vi "EJ 3.3.vi"() -> ()   [LabVIEW 2013]
uses:
  <vilib>/sound2/lvsound2.llb/Sound Input Read (DBL).vi
panel:
  in  "stop":bool
  in  "Cluster":T1
  out "Waveform Graph":dbl[](graph)
  in  "Buffer de lectura":dbl=11025.0
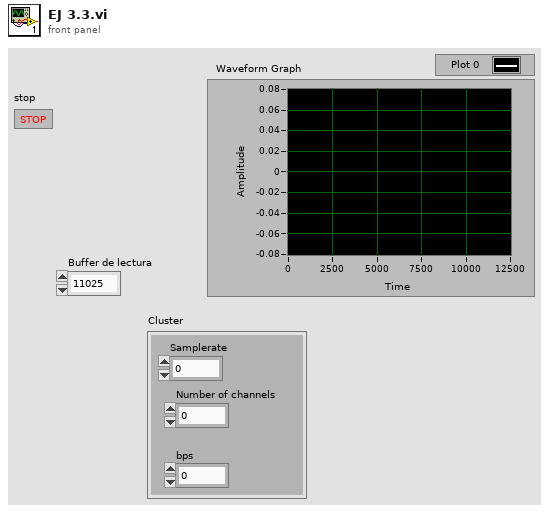
[diagram p1: front panel]
types:
  T1 = cluster{"Samplerate":dbl, "Number of channels":dbl, "bps":dbl}
  T2 = typedef "Sound Input Task ID.ctl" = u32
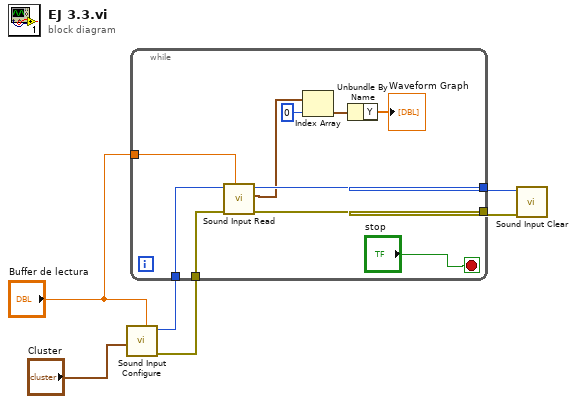
[diagram p0: block diagram]
diagram:
  n1 = call <vilib>:"Sound Input Configure.vi"("number of samples/ch"="Buffer de lectura", "sound format"="Cluster") -> ("error out"=w6:errorcluster, "task ID"=w4:T2)  [unwired: 8 in]
  n2 = while {
    tunnel: w6 -> [w14]
    tunnel: [w13] -> w5
    tunnel: w4 -> [w15]
    tunnel: [w16] -> w3
    tunnel: "Buffer de lectura" -> [w12]
    stop <- "stop" stop-if-true
    n3 = call-poly <vilib>:"Sound Input Read.vi"("number of samples/ch"=w12, "error in (no error)"=w14, "task ID"=w15) -> ("error out"=w13:errorcluster, "data"=w11:waveform(dbl)[], "task ID out"=w16:T2)  [unwired: 6 in]
    n4 = Index Array(array=w11, index=0) -> (element=w9:waveform(dbl))
    n5 = Unbundle By Name(w9) -> ("Y"=→"Waveform Graph":dbl[])
  }
  n6 = call <vilib>:"Sound Input Clear.vi"("error in (no error)"=w5, "task ID"=w3) -> ()  [unwired: 9 in, 1 out]
